vi "DAQ_TRTD Meas Initialize.vi"(0 "Physical Channels":tag, 7 "Global Channels":refnum<k21>, 11 "error in":errorcluster) -> (4 "DAQmx Task Out":refnum<k21>, 15 "error out":errorcluster)   [LabVIEW 2021, in "DAQ_Temperature RTD Measurement.lvlib"]
doc: "Initialize analog input channels for Temperature RTD and obtains a DAQmx task\n\nProvide either Physical channel or Global Channel\nIf both physical and Global channels are provided, Global Channels will take precedence"
uses:
  DAQ_Temperature RTD Measurement.lvlib
  <vilib>/DAQmx/create/channels.llb/DAQmx Create Channel (AI-Temperature-RTD).vi
panel:
  # "Inputs"
  # "Outputs"
  # "Overview:\nThis VI initializes NI cDAQ AI Module and provides the DAQmx Task Out\n\nHardware Requirements: NI C Series/cDAQ Temperature Input Module (Ex: NI-9217)\n\nSoftware Requirements: NI DAQmx 2022 Q4 or later\n\nInstructions:\n1. Enter physical channel in which Temparature Measurement has to be done in Physical Channels control. (Or) Enter Global channels to use it instead of initiating a new task. User must configure only one input. If both are provided, Global Channels will take precedence.\n3. Get the Time Domain Measurement task from DAQmx Task Out\n\nNote: User can use the DAQmx Task on other modules to configure and initiate Temparature RTD Measurements."
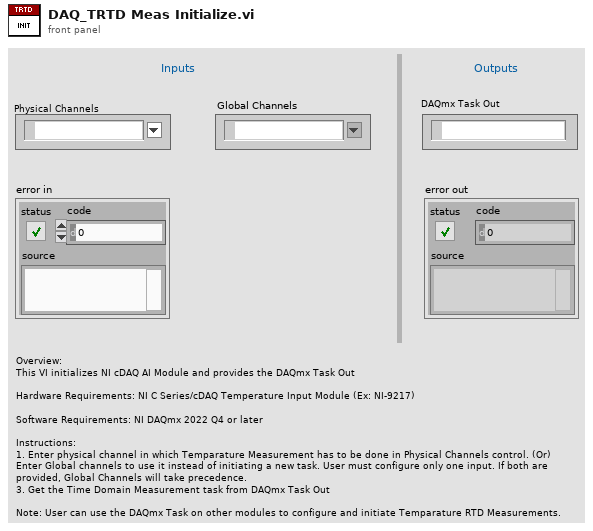
[diagram p1: front panel]
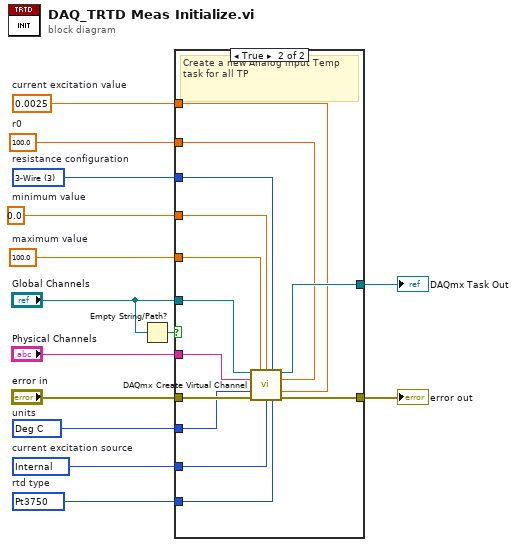
[diagram p0: block diagram]
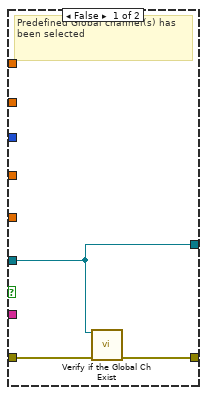
[diagram p2: hidden frame]
diagram:
  w1 = 12481 items=["Pt3750"=12481, "Pt3851"=10071, "Pt3911"=12482, "Pt3916"=10069, "Pt3920"=10053, "Pt3928"=12483, "Custom"=10137]  # rtd type
  w2 = 10200 items=["Internal"=10200, "External"=10167, "None"=10230]  # current excitation source
  w3 = 0.0025  # current excitation value
  w4 = 100.0  # r0
  w5 = 10143 items=["Deg C"=10143, "Deg F"=10144, "Kelvins"=10325, "Deg R"=10145, "From Custom Scale"=10065]  # units
  w6 = 3 items=["2-Wire"=2, "3-Wire"=3, "4-Wire"=4]  # resistance configuration
  w7 = 0.0  # minimum value
  w8 = 100.0  # maximum value
  n1 = Empty String/Path?(string/path="Global Channels") -> (empty?=w10:bool)
  n2 = case shown="True" w10 {
    tunnel: "Physical Channels" -> [_ w27]
    tunnel: "Global Channels" -> [w15 w30]
    tunnel: [w15 w29] -> w11
    tunnel: "error in" -> [w17 w28]
    tunnel: [w16 w26] -> w14
    tunnel: w8 -> [_ w25]
    tunnel: w7 -> [_ w24]
    tunnel: w6 -> [_ w23]
    tunnel: w5 -> [_ w22]
    tunnel: w4 -> [_ w21]
    tunnel: w3 -> [_ w20]
    tunnel: w2 -> [_ w19]
    tunnel: w1 -> [_ w18]
    frame False {
      # "Predefined Global channel(s) has been selected"
      n3 = call "Verify if the Global Ch Exist.vi"("Global Channels"=w15, "error in (no error)"=w17) -> ("error out"=w16:errorcluster)  [unwired: 13 in]
    }
    frame True {
      # "Create a new Analog input Temp task for all TP"
      n4 = call-poly <vilib>:"DAQmx Create Virtual Channel.vi"("task in"=w30, "maximum value"=w25, "minimum value"=w24, "resistance configuration"=w23, "physical channels"=w27, "r0"=w21, "units"=w22, "current excitation value"=w20, "error in"=w28, "current excitation source"=w19, "rtd type"=w18) -> ("task out"=w29:refnum<k21>, "error out"=w26:errorcluster)  [unwired: 3 in]
    }
  }
  "DAQmx Task Out" <- w11
  "error out" <- w14
